vi "Initialise Raw Queue.vi"(8 "error in (no error)":errorcluster) -> (0 "error out":errorcluster)   [LabVIEW 2017]
uses:
  Application Control/Application Globals.vi
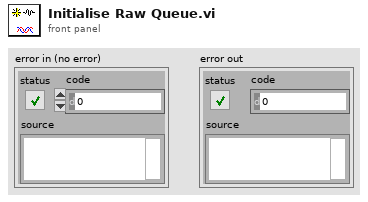
[diagram p1: front panel]
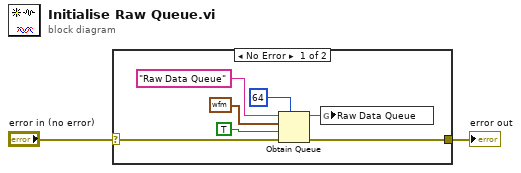
[diagram p0: block diagram]
diagram:
  n1 = case shown="No Error" "error in (no error)" {
    selector: "error in (no error)" -> [w4 w10]
    tunnel: [w3 w10] -> w2
    frame No Error {
      n2 = Obtain Queue(max queue size (-1, unlimited)=64, name (unnamed)="Raw Data Queue", element data type=waveform(cdb) {"t0"=timestamp(0 s since 1904-01-01), "dt"=1.0, "Y"=[]} ("data out"), create if not found? (T)=TRUE, error in (no error)=w4) -> (queue out=w5:refnum<queue>, error out=w3:errorcluster)  [unwired: 1 out]
      n3 = global write "Application Globals.vi" "Raw Data Queue"(w5) -> ()
    }
    frame Error {
    }
  }
  "error out" <- w2
